vi "Write LoopStopCondition.vi"(8 "error in (no error)":errorcluster, 10 "LoopStopCondition":T1, 11 "Test in":refnum<class "Test.lvclass">) -> (0 "error out":errorcluster, 3 "Test out":refnum<class "Test.lvclass">)   [LabVIEW 2014, in "Test.lvclass"]
uses:
  Test.lvclass
  Typedef/LoopStopCondition.ctl
  Test.lvclass/Test.ctl
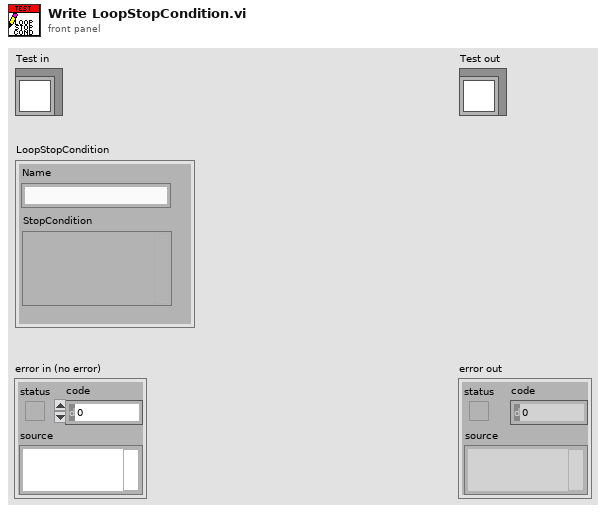
[diagram p1: front panel]
types:
  T1 = typedef "Test.lvclass/LoopStopCondition.ctl" = cluster{"Name":string, "StopCondition":variant}
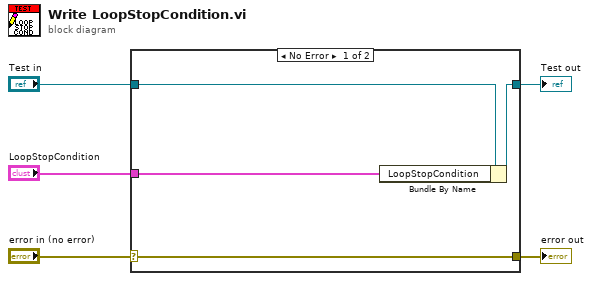
[diagram p0: block diagram]
diagram:
  n1 = case shown="No Error" "error in (no error)" {
    selector: "error in (no error)" -> [w9 w10]
    tunnel: [w9 w10] -> w4
    tunnel: [w7 w11] -> w2
    tunnel: "Test in" -> [w8 w11]
    tunnel: "LoopStopCondition" -> [w6 _]
    frame No Error {
      n2 = Bundle By Name(cluster=w8, "LoopStopCondition"=w6) -> (w7:refnum<class "Test.lvclass">)
    }
    frame Error {
    }
  }
  "error out" <- w4
  "Test out" <- w2
